vi "AS_OUT.vi"(8 "error in (no error)":errorcluster, 9 "拍攝L讀取條碼":string, 10 "拍攝R讀取條碼":string, 11 "DBLink":string) -> (0 "error out":errorcluster, 2 "Workspace: screw_A":cluster{"條碼A":string, "條碼B":string}[](array[cluster]), 3 "Workspace: Assemble":cluster{"條碼A":string, "條碼B":string}[](array[cluster]))   [LabVIEW 2019]
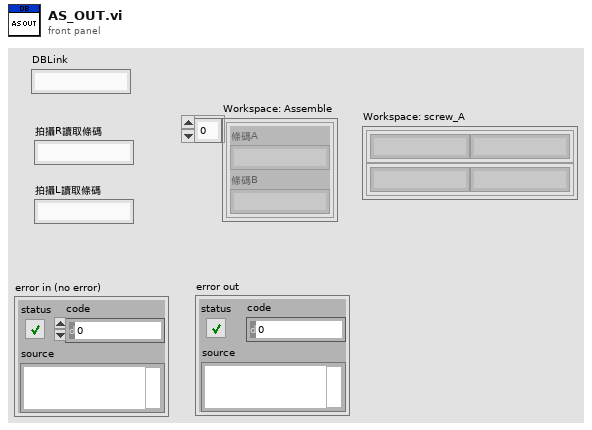
[diagram p1: front panel]
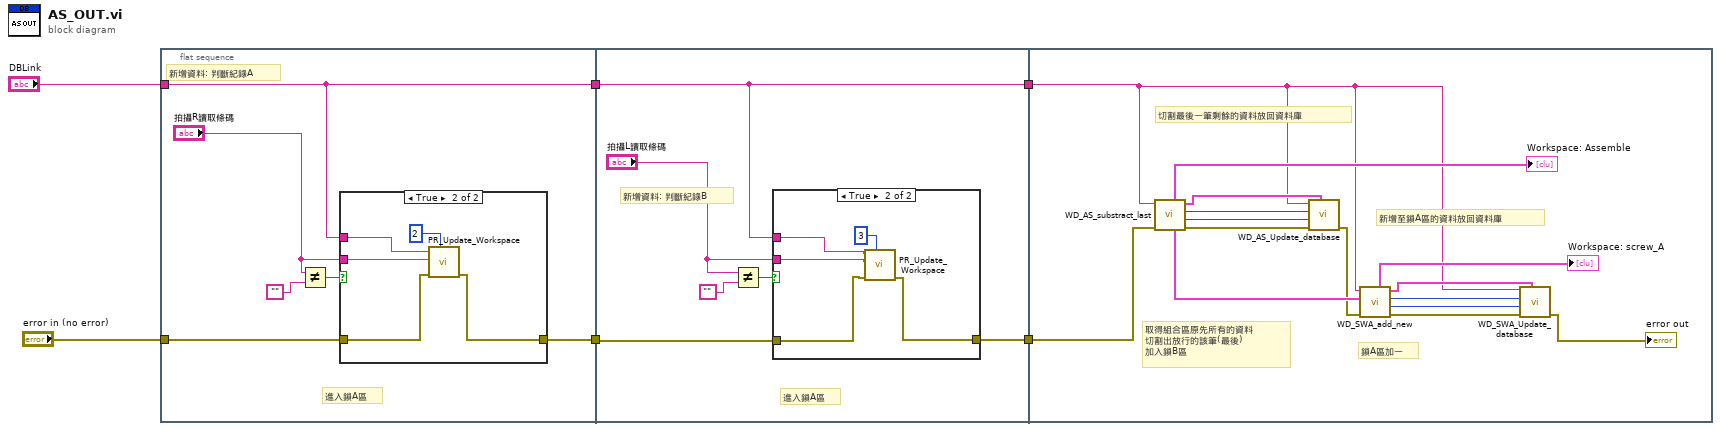
[diagram p0: block diagram]
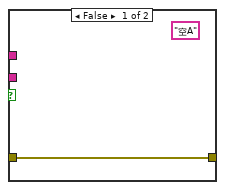
[diagram p2: hidden frame]
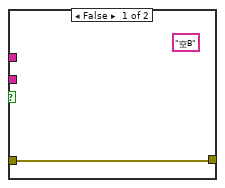
[diagram p3: hidden frame]
diagram:
  n1 = flat-sequence {
    tunnel: "DBLink" -> [w12]
    tunnel: [w12] -> w4
    tunnel: "error in (no error)" -> [w9]
    tunnel: [w8] -> w3
    tunnel: w4 -> [w19]
    tunnel: w3 -> [w21]
    tunnel: [w20] -> w2
    tunnel: [w19] -> w1
    tunnel: w2 -> [w32]
    tunnel: w1 -> [w31]
    frame #0 {
      # "進入鎖A區"
      # "新增資料: 判斷紀錄A"
      n2 = Not Equal?(x="拍攝R讀取條碼", y="") -> (x != y?=w10:bool)
      n3 = case shown="True" w10 {
        tunnel: w12 -> [_ w18]
        tunnel: "拍攝R讀取條碼" -> [_ w17]
        tunnel: w9 -> [w13 w16]
        tunnel: [w13 w14] -> w8
        frame False {
          (unwired) "空A"
        }
        frame True {
          n4 = call "PR_Update_Workspace .vi"("[workplace_id]"=i16 2 ("workspace"), "error in (no error)"=w16, "barcode"=w17, "DBlink"=w18) -> ("error out"=w14:errorcluster)  [unwired: 7 in]
        }
      }
    }
    frame #1 {
      # "進入鎖A區"
      # "新增資料: 判斷紀錄B"
      n5 = Not Equal?(x="拍攝L讀取條碼", y="") -> (x != y?=w23:bool)
      n6 = case shown="True" w23 {
        tunnel: w19 -> [_ w30]
        tunnel: "拍攝L讀取條碼" -> [_ w29]
        tunnel: [w25 w26] -> w20
        tunnel: w21 -> [w25 w28]
        frame False {
          (unwired) "空B"
        }
        frame True {
          n7 = call "PR_Update_Workspace .vi"("[workplace_id]"=i16 3 ("workspace"), "error in (no error)"=w28, "barcode"=w29, "DBlink"=w30) -> ("error out"=w26:errorcluster)  [unwired: 7 in]
        }
      }
    }
    frame #2 {
      # "新增至鎖A區的資料放回資料庫"
      # "切割最後一筆剩餘的資料放回資料庫"
      # "取得組合區原先所有的資料\n切割出放行的該筆(最後)\n加入鎖B區"
      # "鎖A區加一"
      n8 = call "WD_AS_substract_last.vi"("error in (no error)"=w32, "DBLink"=w31) -> ("error out"=w38:errorcluster, "站點總數"=w37:i32, "當前料數"=w36:i32, "計算用 array"=w39:cluster{"條碼A":string, "條碼B":string}[], "取出element"=w40:cluster{"條碼A":string, "條碼B":string}, "顯示用array"=→"Workspace: Assemble":cluster{"條碼A":string, "條碼B":string}[])  [unwired: 4 in]
      n9 = call "WD_AS_Update_database.vi"("計算用array"=w39, "error in (no error)"=w38, "站點總數"=w37, "當前料數"=w36, "DBLink"=w31) -> ("error out"=w34:errorcluster)  [unwired: 6 in]
      n10 = call "WD_SWA_add_new.vi"("error in (no error)"=w34, "New data"=w40, "DBLink"=w31) -> ("error out"=w42:errorcluster, "站點總數"=w43:i32, "當前料數"=w44:i32, "計算用 array"=w45:cluster{"條碼A":string, "條碼B":string}[], "顯示用array"=→"Workspace: screw_A":cluster{"條碼A":string, "條碼B":string}[])  [unwired: 4 in]
      n11 = call "WD_SWA_Update_database.vi"("計算用array"=w45, "error in (no error)"=w42, "站點總數"=w43, "當前料數"=w44, "DBLink"=w31) -> ("error out"=→"error out":errorcluster)  [unwired: 6 in]
    }
  }
